vi "Select Channel.vi"(8 "error in (no error)":errorcluster, 10 "Active Channel":i32, 11 "FunctionGenerator in":refnum<class "FunctionGenerator.lvclass">) -> (0 "error out":errorcluster, 3 "FunctionGenerator out":refnum<class "FunctionGenerator.lvclass">)   [LabVIEW 2019, in "FunctionGenerator.lvlib" / "FunctionGenerator.lvclass"]
uses:
  Library/FunctionGenerator.lvclass
  Library/FunctionGenerator.lvclass/FunctionGenerator.ctl
  builds/Engine/Engine.lvlibp/Project/Engine.lvclass
  C:/Users/Public/Documents/Development/builds/Engine/Engine.lvlibp/Project/Engine.lvclass
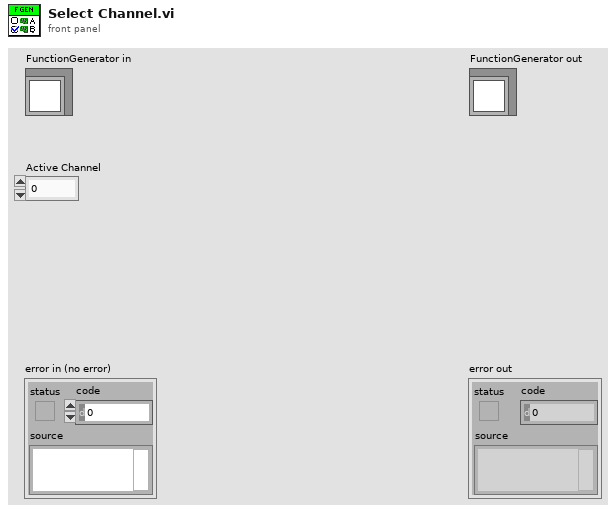
[diagram p1: front panel]
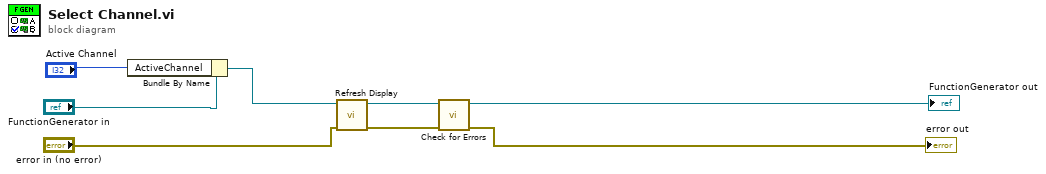
[diagram p0: block diagram]
diagram:
  n1 = Bundle By Name(cluster="FunctionGenerator in", "ActiveChannel"="Active Channel") -> (w6:refnum<class "FunctionGenerator.lvclass">)
  n2 = call "Refresh Display.vi"("error in (no error)"="error in (no error)", "FunctionGenerator in"=w6) -> ("error out"=w4:errorcluster, "FunctionGenerator out"=w2:refnum<class "FunctionGenerator.lvclass">)  [unwired: 8 in]
  n3 = call "Check for Errors.vi"("error in"=w4, "Engine in"=w2) -> ("error out"=→"error out":errorcluster, "Engine out"=→"FunctionGenerator out":refnum<class "FunctionGenerator.lvclass">)  [unwired: 8 in]
